vi "EQ_timeout_autocalcul.vi"(7 "Number of pixels":u32=5 min=1 max=100 step=1, 9 "Chip ID":u32 format="%04x", 10 "Layer ID":u32 format="%04x") -> (2 "EQ timeout auto (s)":u32=1800 caption="Timeout (s)")   [LabVIEW 2015]
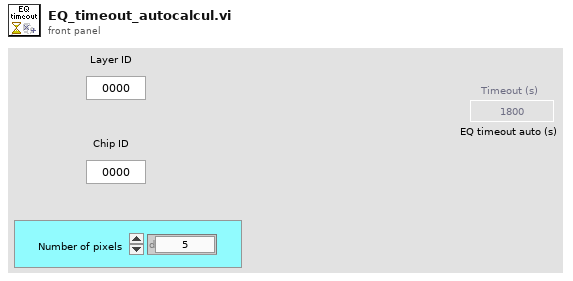
[diagram p1: front panel]
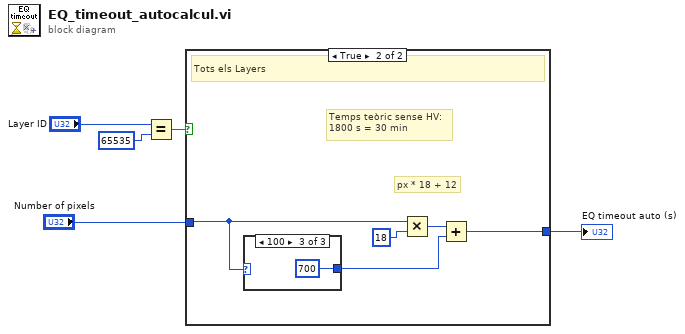
[diagram p0: block diagram]
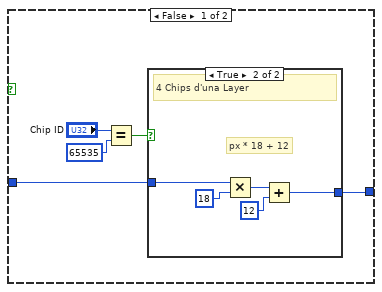
[diagram p2: hidden frame]
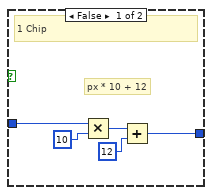
[diagram p3: hidden frame]
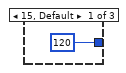
[diagram p4: hidden frame]
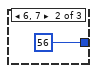
[diagram p5: hidden frame]
diagram:
  n1 = Equal?(x="Layer ID", y=u32 65535 ("Chip ID")) -> (x = y?=w3:bool)
  n2 = case shown="True" w3 {
    tunnel: [w6 w23] -> w1
    tunnel: "Number of pixels" -> [w7 w22]
    frame False {
      n3 = Equal?(x="Chip ID", y=u32 65535 ("Chip ID")) -> (x = y?=w8:bool)
      n4 = case shown="True" w8 {
        tunnel: w7 -> [w15 w17]
        tunnel: [w11 w16] -> w6
        frame False {
          # "px * 10 + 12"
          # "1 Chip"
          n5 = Multiply(x=w15, y=u32 10) -> (x*y=w13:u32)
          n6 = Add(x=w13, y=u32 12) -> (x+y=w11:u32)
        }
        frame True {
          # "px * 18 + 12"
          # "4 Chips d'una Layer"
          n7 = Multiply(x=w17, y=u32 18) -> (x*y=w19:u32)
          n8 = Add(x=w19, y=u32 12) -> (x+y=w16:u32)
        }
      }
    }
    frame True {
      # "Temps teòric sense HV:\n1800 s = 30 min"
      # "px * 18 + 12"
      # "Tots els Layers"
      n9 = case shown="100" w22 {
        tunnel: [u32 120 ("y") u32 56 ("y") u32 700 ("y")] -> w21
        frame 15, Default {
        }
        frame 6, 7 {
        }
        frame 100 {
        }
      }
      n10 = Multiply(x=w22, y=u32 18) -> (x*y=w24:u32)
      n11 = Add(x=w24, y=w21) -> (x+y=w23:u32)
    }
  }
  "EQ timeout auto (s)" <- w1
